vi "Read_XML_CIACS.vi"(3 "ReferenceToControl":refnum<vi>, 5 "XML_Cluster_String":string) -> (0 "Name":string, 1 "type":string, 2 "before match":string, 6 "Array":string[](array[string]))   [LabVIEW 2011]
uses:
  <vilib>/INL/TimMcJLabviewUtilities/XML_File_Control_Read/Read_XLM_lib.lvlib
panel:
  out "Numeric 2":i32
  out "stripped Cluster":string
  out "Cluster_string":string
  out "remaining":string
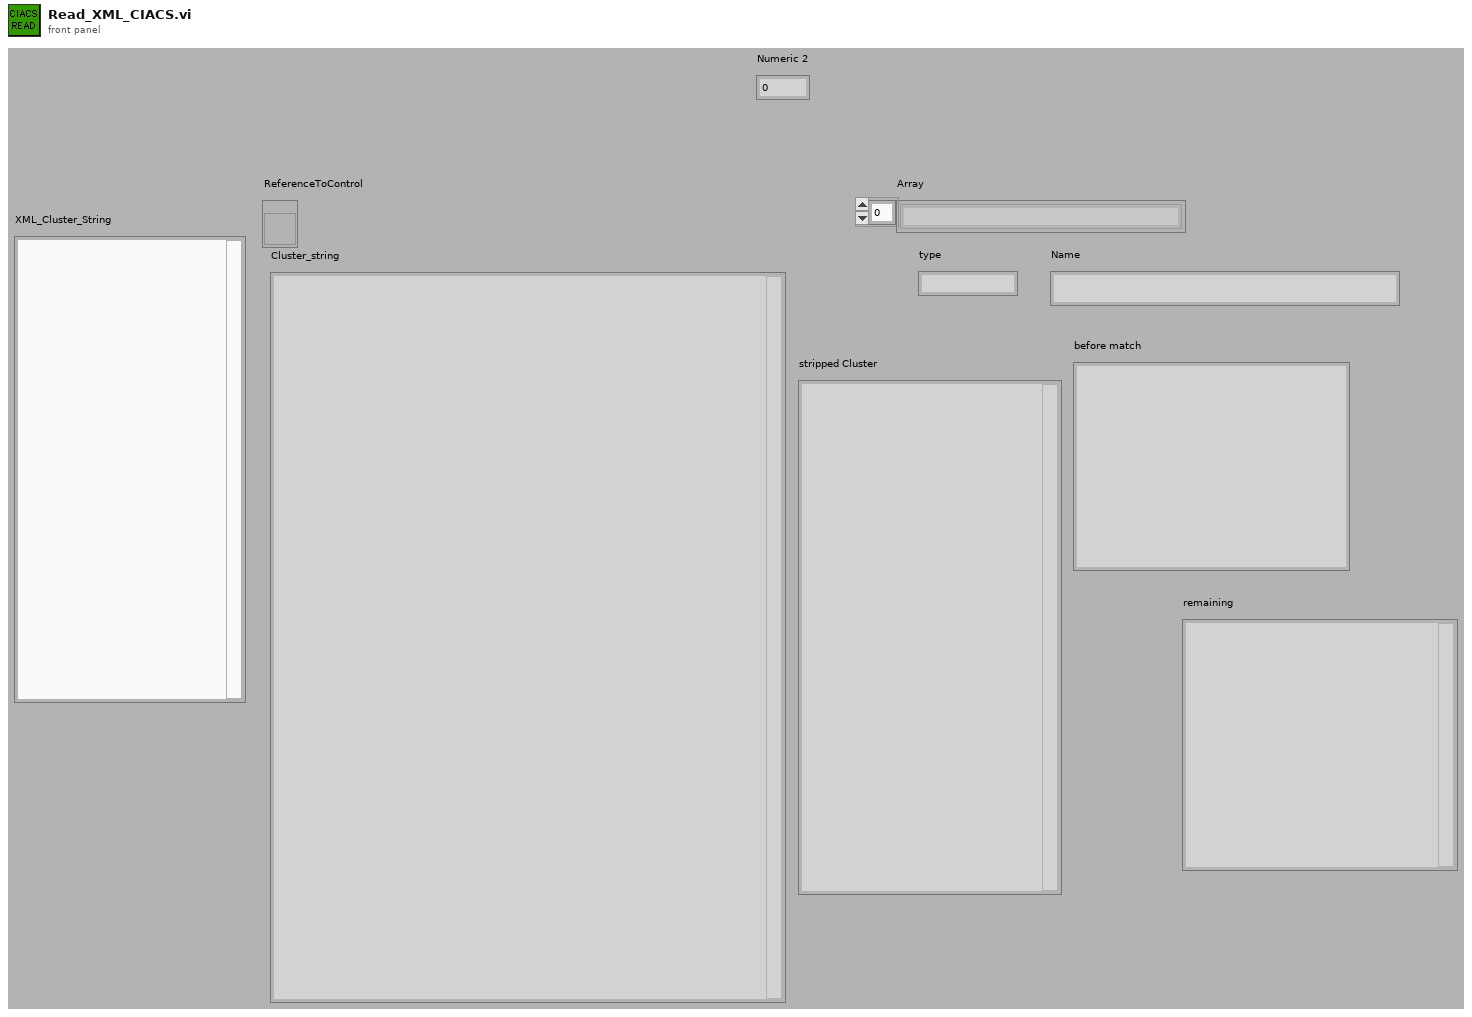
[diagram p1: front panel]
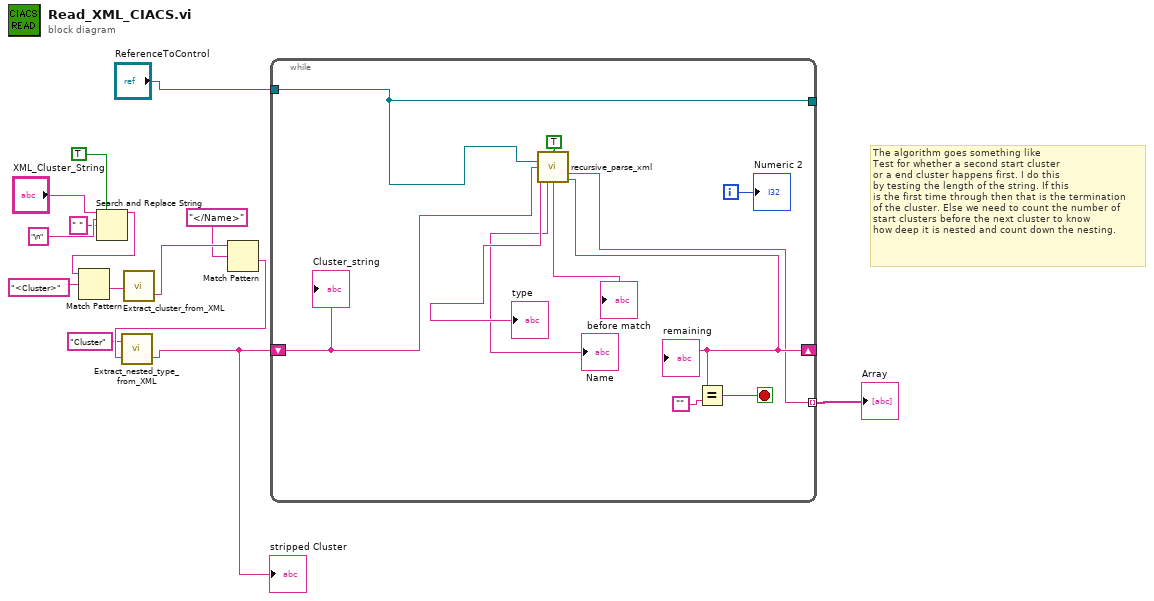
[diagram p0: block diagram]
diagram:
  # "The algorithm goes something like\nTest for whether a second start cluster\nor a end cluster happens first. I do this \nby testing the length of the string. If this\nis the first time through then that is the termination\nof the cluster. Else we need to count the number of\nstart clusters before the next cluster to know\nhow deep it is nested and count down the nesting."
  n1 = Search and Replace String(replace all?=TRUE ("replace all? (F)"), input string="XML_Cluster_String", search string="\n", replace string=" " ("replace string (\"\")")) -> (result string=w2:string)  [unwired: 4 in, 3 out]
  n2 = Match Pattern(string=w2, regular expression="<Cluster>") -> (after substring=w11:string)  [unwired: 1 in, 3 out]
  n3 = call "Extract_cluster_from_XML.vi"("XML_Cluster_String"=w11) -> ("Cluster"=w8:string)  [unwired: 1 out]
  n4 = Match Pattern(string=w8, regular expression="</Name>") -> (after substring=w6:string)  [unwired: 1 in, 3 out]
  n5 = call <vilib>:"Extract_nested_type_from_XML.vi"("XML_Cluster_String"=w6, "type"="Cluster") -> ("Cluster"=w4:string)  [unwired: 1 out]
  "stripped Cluster" <- w4
  n6 = while {
    shift-right: [w16] -> _
    shift-left: w4 -> [w20]
    tunnel: [w15] -> w14 mode=indexing
    tunnel: "ReferenceToControl" -> [w22]
    tunnel: [w22] -> _
    i -> [w23]
    stop <- w24 stop-if-true
    n7 = call "recursive_parse_xml.vi"("Is_Cluster"=TRUE, "Input_reference"=w22, "Input_XML"=w20) -> ("After_cluster"=w15:string, "DataType_name"=→"type":string, "Name"=→"Name":string, "before name match"=→"before match":string, "remaining XML string"=w16:string)  [unwired: 5 in, 3 out]
    "remaining" <- w16
    n8 = Equal?(x=w16, y="") -> (x = y?=w24:bool)
    "Cluster_string" <- w20
    "Numeric 2" <- w23
  }
  "Array" <- w14
